vi "emi_Read Key Anything.vi"(0 "Ini file refnum":T1, 1 "Section(Default)":string="Default", 5 "Name":string, 7 "Anything":variant, 11 "error in (no error)":errorcluster) -> (4 "Ini file refnum out":T1, 8 "Anything Out":variant, 14 "Found":bool, 15 "error out":errorcluster)   [LabVIEW 2011]
doc: "Use in the same way as Read key. Anything in may contain a cluster.\nAny data wired to Anything must be named, that includes any item in a cluster.\nThis is a slow VI, keep in mind when desiding where to use.\n\nINEGN ARRAY SUPPORT\n\nThe cluster can contain anything(Including other clusters) except:\nARRAY\nVariant\nPicture\nTag\nWaveform\nDigital Waveform\nDigital Data\nExpressData\nRefnum\nExternal Data\nVI\nPoly VI\nLabview Class Instance\nFixed point"
uses:
  <vilib>/Utility/config.llb/Config Data RefNum.ctl
  Error/emi_Create Error.vi
  <vilib>/Utility/config.llb/Read Key (String).vi
  <vilib>/Utility/VariantDataType/GetNumericInfo.vi
  <vilib>/Utility/VariantDataType/SetTypeInfo.vi
  <vilib>/Utility/error.llb/Trim Whitespace.vi
  <vilib>/Utility/VariantDataType/SetNumericInfo.vi
  <vilib>/Utility/VariantDataType/VariantType.lvlib
  <vilib>/Utility/config.llb/NI_LVConfig.lvlib
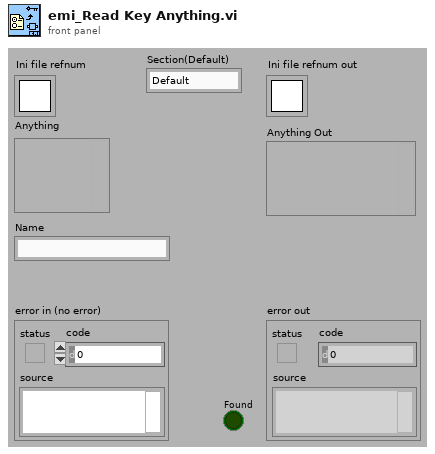
[diagram p1: front panel]
types:
  T1 = typedef "NI_LVConfig.lvlib/Config Data RefNum.ctl" = refnum<k1>
  T2 = typedef "VariantType.lvlib/Type.ctl" = enum8{"Invalid Type", "Void", "I8", "I16", "I32", "I64", "U8", "U16", "U32", "U64", "Single Float", "Double Float", "Extended Float", "Single Complex", "Double Complex", "Extended Complex", "Enum U8", "Enum U16", "Enum U32", "Enum U64", "Single Float With Unit", "Double Float With Unit", "Extended Float With Unit", "Single Complex with Unit", "Double Complex with Unit", "Extended Complex with Unit", "Boolean", "String", "Path", "Picture", "Tag", "Array", "Cluster", "Variant", "LV Variant", "Waveform", "Timestamp", "Digital Waveform", "Digital Data", "ExpressData", "Refnum", "External Data", "VI", "Poly VI", "LabVIEW Class Instance", "Fixed Point"}
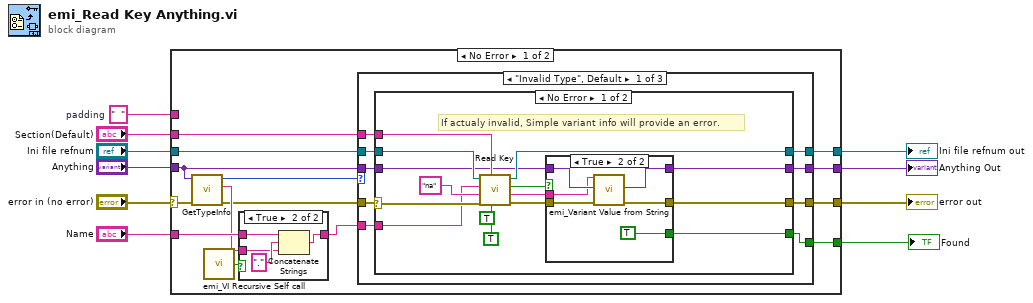
[diagram p0: block diagram]
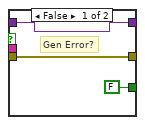
[diagram p2: hidden frame]
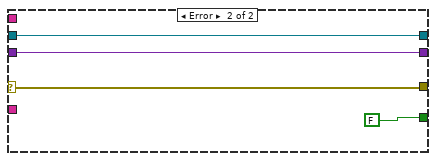
[diagram p3: hidden frame]
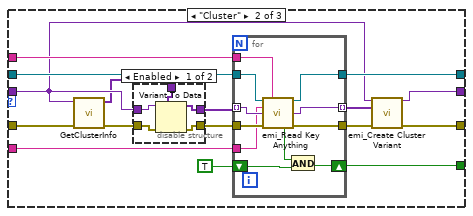
[diagram p4: hidden frame]
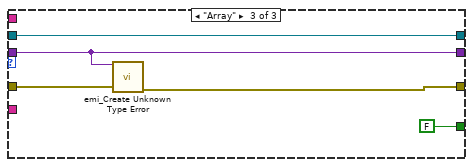
[diagram p6: hidden frame]
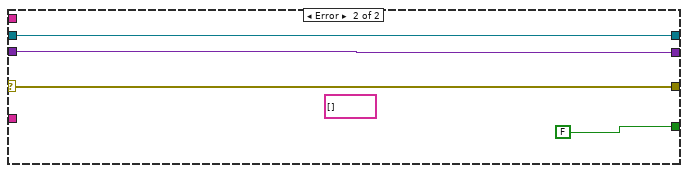
[diagram p8: hidden frame]
diagram:
  w5 = "  "  # padding
  n1 = case shown="No Error" "error in (no error)" {
    selector: "error in (no error)" -> [w24 w108]
    tunnel: "Anything" -> [w18 w106]
    tunnel: [w15 w108] -> w8
    tunnel: "Name" -> [w22 _]
    tunnel: "Ini file refnum" -> [w17 w107]
    tunnel: "Section(Default)" -> [w16 _]
    tunnel: w5 -> [_ _]
    tunnel: [w14 w107] -> w4
    tunnel: [w13 w106] -> w3
    tunnel: [w11 FALSE ("Found")] -> w1
    frame No Error {
      n2 = call <vilib>:"GetTypeInfo.vi"("error in (no error)"=w24, "Variant"=w18) -> ("error out"=w20:errorcluster, "Name"=w21:string, "Type Enum"=w19:T2)  [unwired: 5 in, 2 out]
      n3 = call "emi_VI Recursive Self call.vi"() -> ("Recursive Self Call?"=w23:bool)  [unwired: 15 in]
      n4 = case shown="True" w23 {
        tunnel: [w100 w103] -> w12
        tunnel: w22 -> [w100 w102]
        tunnel: w21 -> [_ w101]
        frame False {
        }
        frame True {
          n5 = Concatenate Strings(w102, "." ("string"), w101) -> (w103:string)
        }
      }
      n6 = case shown="\"Invalid Type\", Default" w19 {
        tunnel: w18 -> [w28 w66 w96]
        tunnel: w20 -> [w30 w72 w98]
        tunnel: [w29 w68 w97] -> w15
        tunnel: w12 -> [w27 w74 _]
        tunnel: w16 -> [w32 w75 _]
        tunnel: w17 -> [w33 w76 w99]
        tunnel: [w31 w73 w99] -> w14
        tunnel: [w26 w69 w96] -> w13
        tunnel: [w25 w62 FALSE ("Found")] -> w11
        frame "Invalid Type", Default {
          n7 = case shown="No Error" w30 {
            selector: w30 -> [w44 w60]
            tunnel: [w41 w60] -> w29
            tunnel: w33 -> [w47 w59]
            tunnel: w27 -> [w36 _]
            tunnel: w32 -> [w46 _]
            tunnel: [w45 w59] -> w31
            tunnel: w28 -> [w40 w58]
            tunnel: [w38 w58] -> w26
            tunnel: [w34 FALSE] -> w25
            frame No Error {
              (unwired) TRUE ("write raw string? (F)")
              # "If actualy invalid, Simple variant info will provide an error."
              n8 = call-poly <vilib>:"Read Key.vi"("read raw string? (F)"=TRUE, "section"=w46, "error in (no error)"=w44, "default value"="na", "key"=w36, "refnum"=w47) -> ("error out"=w42:errorcluster, "value"=w35:string, "found?"=w39:bool, "refnum out"=w45:T1)  [unwired: 2 in]
              n9 = case shown="True" w39 {
                tunnel: w42 -> [w50 w56]
                tunnel: [w50 w55] -> w41
                tunnel: w35 -> [_ w52]
                tunnel: w40 -> [w49 w54]
                tunnel: [w49 w53] -> w38
                tunnel: [FALSE TRUE] -> w34
                frame False {
                  # "Gen Error?"
                }
                frame True {
                  n10 = call "emi_Variant Value from String.vi"("Value"=w52, "Anything"=w54, "error in(no error)"=w56) -> ("Anything & Value"=w53:variant, "error out"=w55:errorcluster)  [unwired: 11 in]
                }
              }
            }
            frame Error {
            }
          }
        }
        frame "Cluster" {
          n11 = call <vilib>:"GetClusterInfo.vi"("error in (no error)"=w72, "Variant"=w66) -> ("error out"=w67:errorcluster, "Cluster Elements"=w65:variant[])  [unwired: 8 in]
          n12 = disable-structure shown="Enabled" {
            disable-tunnel: w67 -> [w81 w83]
            disable-tunnel: w66 -> [w80 _]
            disable-tunnel: w65 -> [w79 w82]
            disable-tunnel: [w78 w83] -> w64
            disable-tunnel: [w77 w82] -> w63
            frame Enabled {
              n13 = Variant To Data(error in=w81, type=w79, Variant=w80) -> (data=w77:variant[], error out=w78:errorcluster)
            }
            frame Disabled {
            }
          }
          n14 = for {
            tunnel: w63 -> [w88] mode=indexing
            tunnel: w64 -> [w94]
            tunnel: [w93] -> w70
            tunnel: w74 -> [w87]
            tunnel: w76 -> [w92]
            tunnel: w75 -> [w91]
            tunnel: [w90] -> w73
            tunnel: [w89] -> w71 mode=indexing
            shift-right: [w85] -> w62
            shift-left: TRUE ("Found") -> [w84]
            n15 = call "emi_Read Key Anything.vi"("Ini file refnum"=w92, "Section(Default)"=w91, "Name"=w87, "Anything"=w88, "error in (no error)"=w94) -> ("Ini file refnum out"=w90:T1, "Anything Out"=w89:variant, "Found"=w86:bool, "error out"=w93:errorcluster)  [unwired: 7 in]
            n16 = And(x=w86, y=w84) -> (x .and. y?=w85:bool)
          }
          n17 = call "emi_Create Cluster Variant.vi"("Cluster"=w66, "Cluster Elements"=w71, "error in (no error)"=w70) -> ("Cluster Out"=w69:variant, "error out"=w68:errorcluster)  [unwired: 11 in]
        }
        frame "Array" {
          n18 = call "emi_Create Unknown Type Error.vi"("Anything"=w96, "error IO"=w98) -> ("error out"=w97:errorcluster)  [unwired: 13 in]
        }
      }
    }
    frame Error {
      (unwired) string[] []
    }
  }
  "error out" <- w8
  "Ini file refnum out" <- w4
  "Anything Out" <- w3
  "Found" <- w1
